vi "AndorCameraSwitch.vi"(8 "error in (no error)":errorcluster, 10 "Andor Camera":bool, 11 "HWConfiguration in":refnum<class "HWConfiguration.lvclass">) -> (0 "error out":errorcluster, 3 "HWConfiguration out":refnum<class "HWConfiguration.lvclass">)   [LabVIEW 2011, in "Hardware.lvlib" / "HWControllers.lvlib" / "HWConfiguration.lvclass"]
uses:
  HWConfiguration.lvclass
  HWConfiguration.lvclass/HWConfiguration.ctl
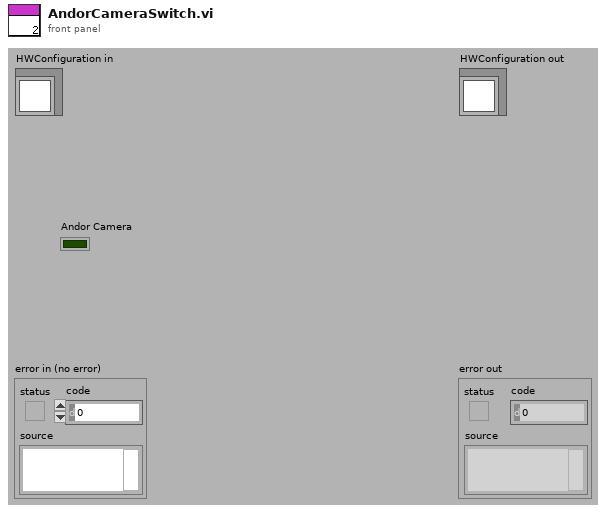
[diagram p1: front panel]
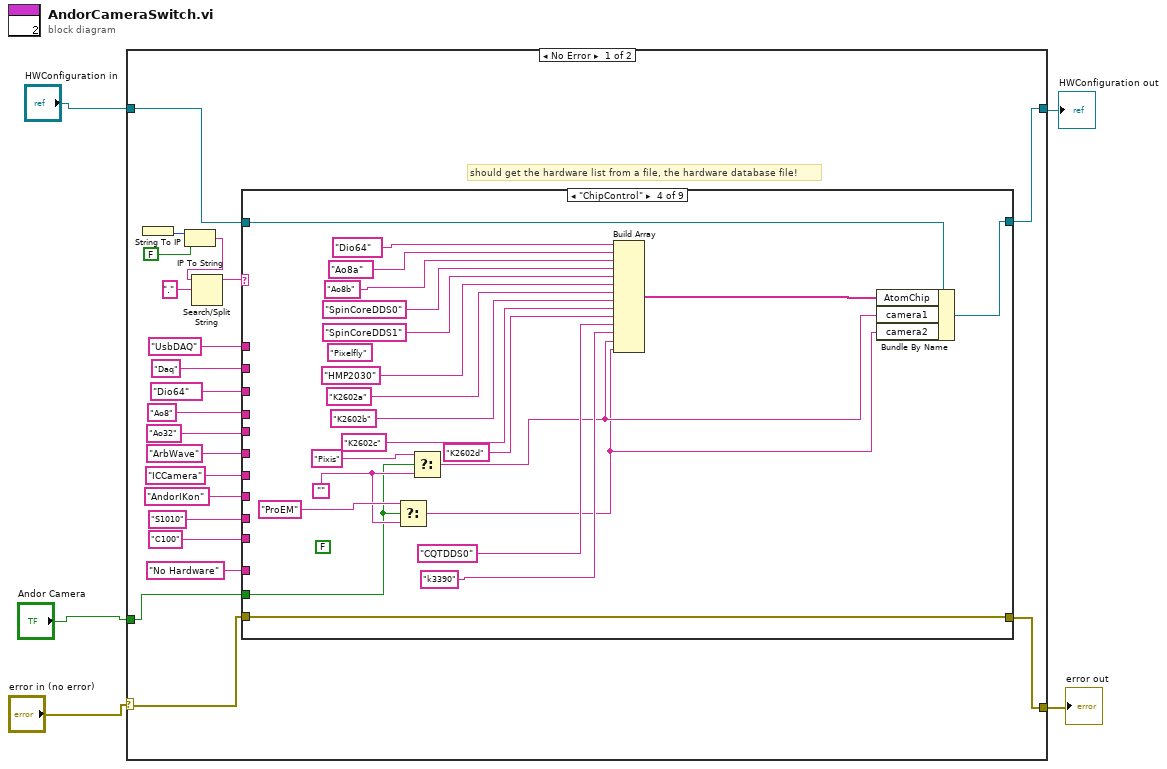
[diagram p0: block diagram]
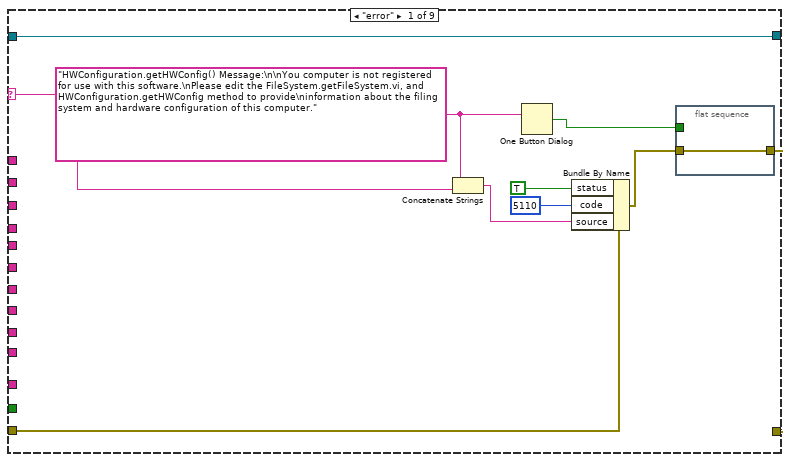
[diagram p2: hidden frame]
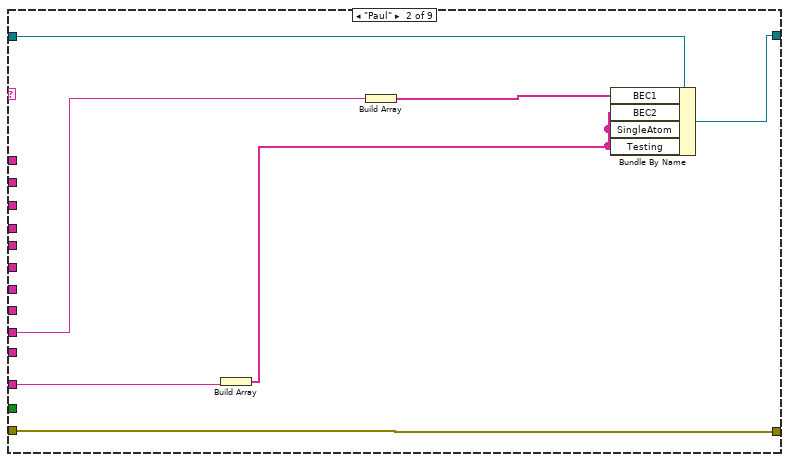
[diagram p3: hidden frame]
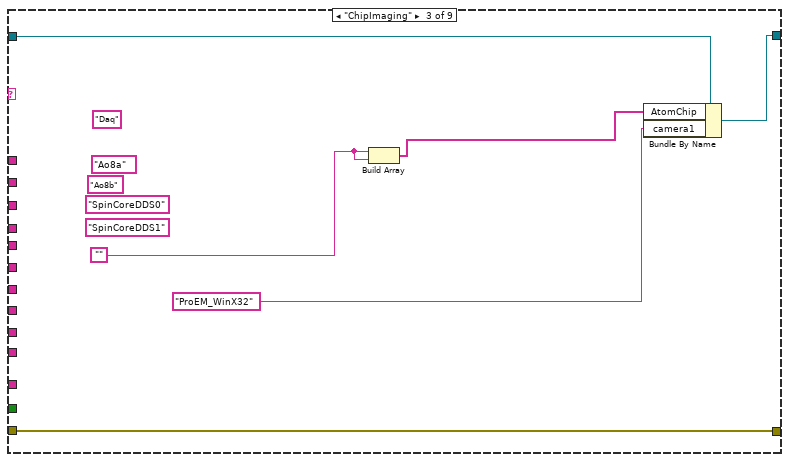
[diagram p4: hidden frame]
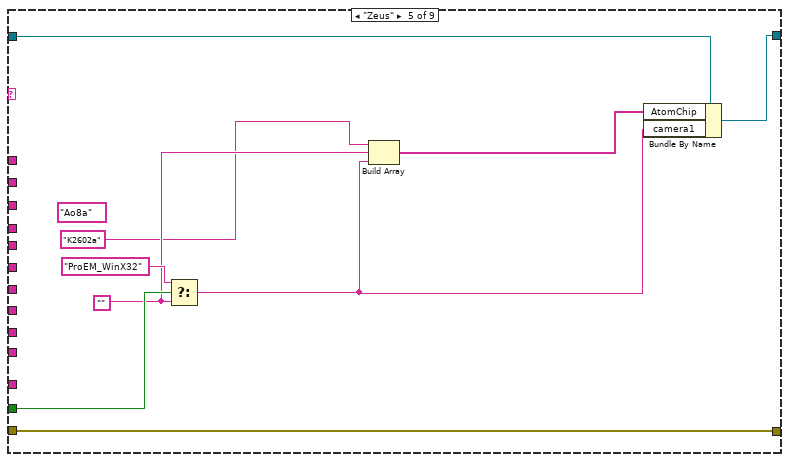
[diagram p5: hidden frame]
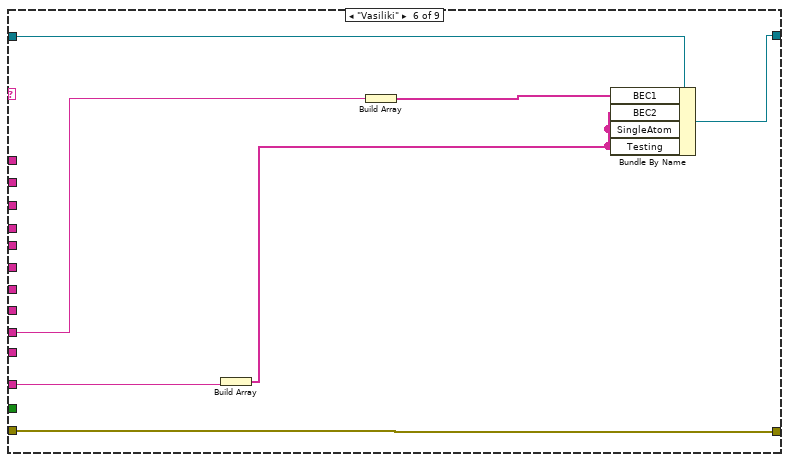
[diagram p6: hidden frame]
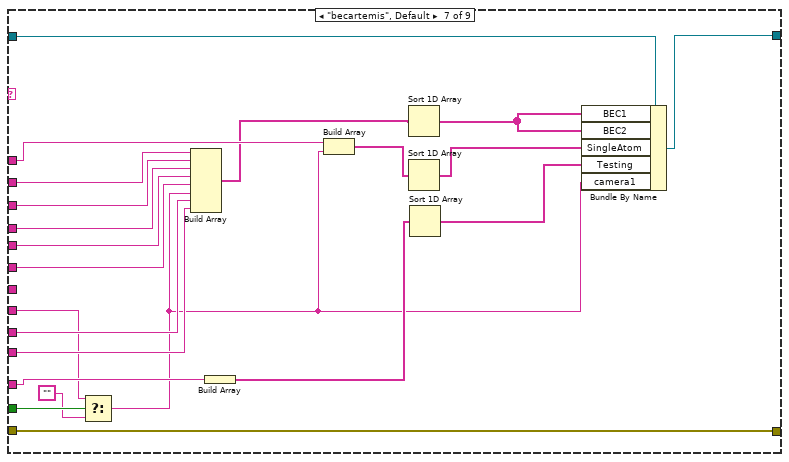
[diagram p7: hidden frame]
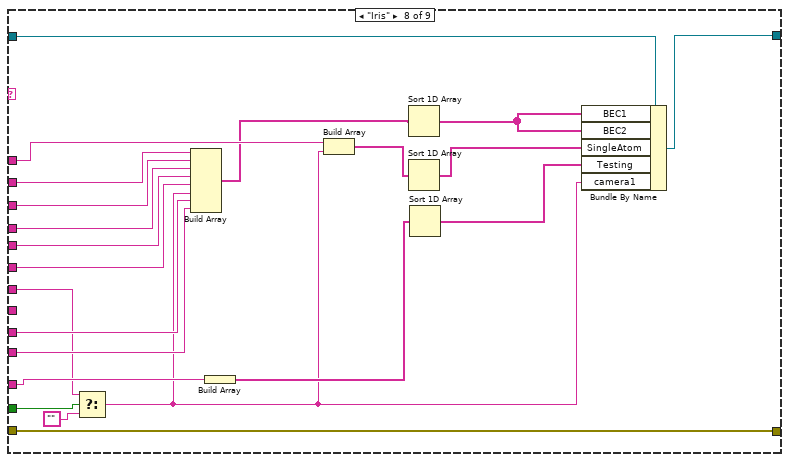
[diagram p8: hidden frame]
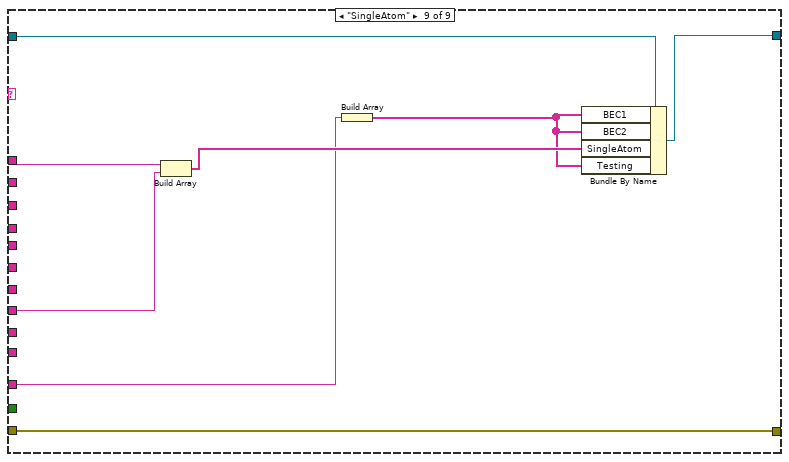
[diagram p9: hidden frame]
diagram:
  n1 = case shown="No Error" "error in (no error)" {
    selector: "error in (no error)" -> [w21 w142]
    tunnel: [w18 w142] -> w3
    tunnel: [w19 w141] -> w2
    tunnel: "HWConfiguration in" -> [w20 w141]
    tunnel: "Andor Camera" -> [w6 _]
    frame No Error {
      # "should get the hardware list from a file, the hardware database file!"
      n2 = String To IP() -> (0:w25:u32)  [unwired: 1 in]
      n3 = IP To String(1:FALSE, 2:w25) -> (0:w23:string)
      n4 = Search/Split String(string=w23, search string/char (-)=".") -> (substring before match=w22:string)  [unwired: 1 in, 2 out]
      n5 = case shown="\"ChipControl\"" w22 {
        selector: w22 -> [w30 _ _ _ _ _ _ _ _]
        tunnel: w20 -> [w27 w43 w50 w72 w81 w87 w109 w131 w139]
        tunnel: [w27 w42 w48 w70 w79 w86 w108 w130 w138] -> w19
        tunnel: w21 -> [w28 w44 w47 w69 w78 w88 w110 w132 w140]
        tunnel: [w33 w44 w47 w69 w78 w88 w110 w132 w140] -> w18
        tunnel: "UsbDAQ" -> [_ _ _ _ _ _ w100 w122 w137]
        tunnel: "Daq" -> [_ _ _ _ _ _ w107 w129 _]
        tunnel: "Dio64" -> [_ _ _ _ _ _ w93 w115 _]
        tunnel: "Ao8" -> [_ _ _ _ _ _ w106 w128 _]
        tunnel: "Ao32" -> [_ _ _ _ _ _ w105 w127 _]
        tunnel: "ArbWave" -> [_ _ _ _ _ _ w104 w126 _]
        tunnel: "ICCamera" -> [_ _ _ _ _ _ _ w112 _]
        tunnel: "AndorIKon" -> [_ _ _ _ _ _ w91 _ w136]
        tunnel: "S1010" -> [_ w39 _ _ _ w83 w103 w125 _]
        tunnel: "C100" -> [_ _ _ _ _ _ w102 w124 _]
        tunnel: "No Hardware" -> [_ w41 _ _ _ w85 w101 w123 w133]
        tunnel: w6 -> [_ _ _ w54 w77 _ w92 w114 _]
        frame "error" {
          w31 = "HWConfiguration.getHWConfig() Message:\n\nYou computer is not registered for use with this software.\nPlease edit the FileSystem.getFileSystem.vi, and HWConfiguration.getHWConfig method to provide\ninformation about the filing system and hardware configuration of this computer."
          n6 = Concatenate Strings(w31, w30) -> (w29:string)
          n7 = One Button Dialog(message=w31) -> (true=w32:bool)  [unwired: 1 in]
          n8 = Bundle By Name(cluster=w28, "status"=TRUE, "code"=5110, "source"=w29) -> (w34:errorcluster)
          n9 = flat-sequence {
            tunnel: w34 -> [w37]
            tunnel: [w37] -> w33
            tunnel: w32 -> [_]
            frame #0 {
            }
          }
        }
        frame "Paul" {
          n10 = Build Array(w41) -> (w40:string[])
          n11 = Build Array(w39) -> (w38:string[])
          n12 = Bundle By Name(cluster=w43, "BEC1"=w38, "BEC2"=w40, "SingleAtom"=w40, "Testing"=w40) -> (w42:refnum<class "HWConfiguration.lvclass">)
        }
        frame "ChipImaging" {
          w46 = ""
          (unwired) "SpinCoreDDS1"
          (unwired) "SpinCoreDDS0"
          (unwired) "Ao8b"
          (unwired) "Ao8a"
          (unwired) "Daq"
          n13 = Build Array(w46, w46) -> (w49:string[])
          n14 = Bundle By Name(cluster=w50, "AtomChip"=w49, "camera1"="ProEM_WinX32") -> (w48:refnum<class "HWConfiguration.lvclass">)
        }
        frame "ChipControl" {
          (unwired) FALSE
          (unwired) "Pixelfly"
          w56 = ""
          n15 = Select(t="ProEM", s=w54, f=w56) -> (s? t:f=w57:string)
          n16 = Select(t="Pixis", s=w54, f=w56) -> (s? t:f=w62:string)
          n17 = Build Array("Dio64", "Ao8a", "Ao8b", "SpinCoreDDS0", "SpinCoreDDS1", "HMP2030", "K2602a", "K2602b", "K2602c", "K2602d", "CQTDDS0", "k3390", w62, w57) -> (w71:string[])
          n18 = Bundle By Name(cluster=w72, "AtomChip"=w71, "camera1"=w62, "camera2"=w57) -> (w70:refnum<class "HWConfiguration.lvclass">)
        }
        frame "Zeus" {
          (unwired) "Ao8a"
          w74 = ""
          n19 = Select(t="ProEM_WinX32", s=w77, f=w74) -> (s? t:f=w76:string)
          n20 = Build Array("K2602a", w74, w76) -> (w80:string[])
          n21 = Bundle By Name(cluster=w81, "AtomChip"=w80, "camera1"=w76) -> (w79:refnum<class "HWConfiguration.lvclass">)
        }
        frame "Vasiliki" {
          n22 = Build Array(w85) -> (w84:string[])
          n23 = Build Array(w83) -> (w82:string[])
          n24 = Bundle By Name(cluster=w87, "BEC1"=w82, "BEC2"=w84, "SingleAtom"=w84, "Testing"=w84) -> (w86:refnum<class "HWConfiguration.lvclass">)
        }
        frame "becartemis", Default {
          n25 = Select(t=w91, s=w92, f="") -> (s? t:f=w89:string)
          n26 = Build Array(w107, w93, w106, w105, w104, w89, w103, w102) -> (w99:string[])
          n27 = Build Array(w101) -> (w95:string[])
          n28 = Build Array(w100, w89) -> (w97:string[])
          n29 = Sort 1D Array(array=w99) -> (sorted array=w98:string[])
          n30 = Sort 1D Array(array=w97) -> (sorted array=w96:string[])
          n31 = Sort 1D Array(array=w95) -> (sorted array=w94:string[])
          n32 = Bundle By Name(cluster=w109, "BEC1"=w98, "BEC2"=w98, "SingleAtom"=w96, "Testing"=w94, "camera1"=w89) -> (w108:refnum<class "HWConfiguration.lvclass">)
        }
        frame "Iris" {
          n33 = Select(t=w112, s=w114, f="") -> (s? t:f=w111:string)
          n34 = Build Array(w129, w115, w128, w127, w126, w111, w125, w124) -> (w121:string[])
          n35 = Build Array(w123) -> (w117:string[])
          n36 = Build Array(w122, w111) -> (w119:string[])
          n37 = Sort 1D Array(array=w121) -> (sorted array=w120:string[])
          n38 = Sort 1D Array(array=w119) -> (sorted array=w118:string[])
          n39 = Sort 1D Array(array=w117) -> (sorted array=w116:string[])
          n40 = Bundle By Name(cluster=w131, "BEC1"=w120, "BEC2"=w120, "SingleAtom"=w118, "Testing"=w116, "camera1"=w111) -> (w130:refnum<class "HWConfiguration.lvclass">)
        }
        frame "SingleAtom" {
          n41 = Build Array(w137, w136) -> (w135:string[])
          n42 = Build Array(w133) -> (w134:string[])
          n43 = Bundle By Name(cluster=w139, "BEC1"=w134, "BEC2"=w134, "SingleAtom"=w135, "Testing"=w134) -> (w138:refnum<class "HWConfiguration.lvclass">)
        }
      }
    }
    frame Error {
    }
  }
  "error out" <- w3
  "HWConfiguration out" <- w2
